vi "GetInt8.vi"(8 "error in (no error)":errorcluster, 11 "MsgPackDeserializer in":refnum<class "MsgPackDeserializer.lvclass">) -> (0 "error out":errorcluster, 2 "Number":i8, 3 "MsgPackDeserializer out":refnum<class "MsgPackDeserializer.lvclass">)   [LabVIEW 2015, in "MsgPackDeserializer.lvclass"]
uses:
  MsgPackDeserializer.lvclass
  MsgPackDeserializer.lvclass/MsgPackDeserializer.ctl
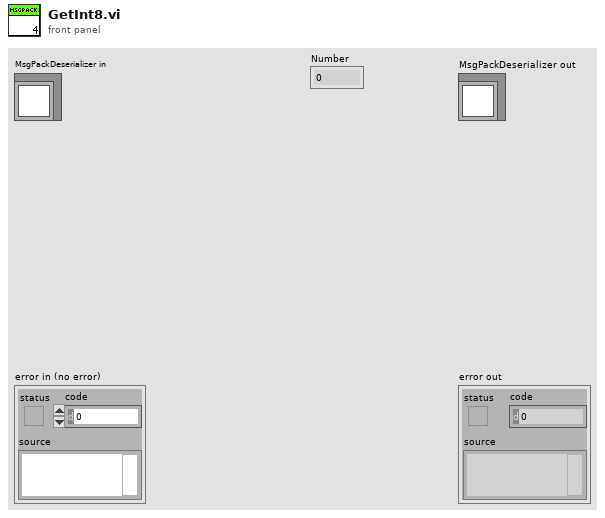
[diagram p1: front panel]
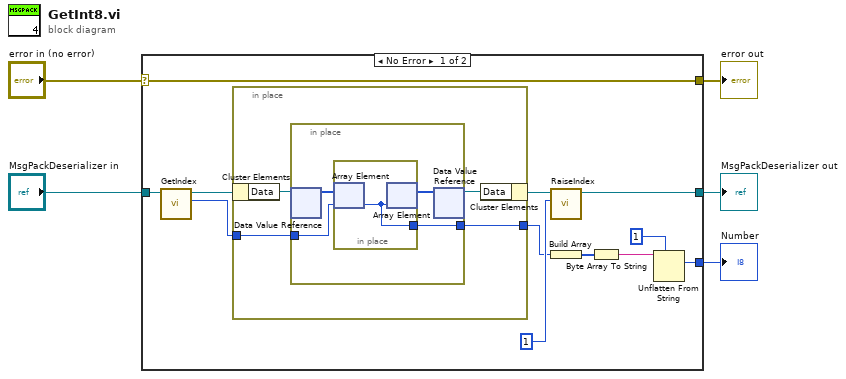
[diagram p0: block diagram]
diagram:
  n1 = case shown="No Error" "error in (no error)" {
    selector: "error in (no error)" -> [w17 w28]
    tunnel: [w17 w28] -> w4
    tunnel: [w13 w27] -> w2
    tunnel: "MsgPackDeserializer in" -> [w16 w27]
    tunnel: [w6 _] -> w1
    frame No Error {
      n2 = call "GetIndex.vi"("MsgPackDeserializer in"=w16) -> ("Index"=w14:i64, "MsgPackDeserializer out"=w15:refnum<class "MsgPackDeserializer.lvclass">)  [unwired: 8 in, 1 out]
      n3 = in-place {
        in-place-border: [w20] -> w10
        in-place-border: w14 -> [w19]
        n4 = in-place-cluster #1(w15) -> ("Data"=w18:refnum<data-value>)
        n5 = in-place {
          in-place-border: [w25] -> w20
          in-place-border: w19 -> [w24]
          n6 = in-place-dvr #2(w18) -> (w23:u8[])  [unwired: 1 out]
          n7 = in-place {
            in-place-border: [w26] -> w25
            n8 = in-place-array #3(w23, w24) -> (w26:u8)
            n9 = in-place-array #3(w26) -> (w22:u8[])  [unwired: 1 out]
          }
          n10 = in-place-dvr #2(w22) -> (w21:refnum<data-value>)  [unwired: 1 out]
        }
        n11 = in-place-cluster #1("Data"=w21) -> (w12:refnum<class "MsgPackDeserializer.lvclass">)
      }
      n12 = call "RaiseIndex.vi"("x"=i64 1, "MsgPackDeserializer in"=w12) -> ("MsgPackDeserializer out"=w13:refnum<class "MsgPackDeserializer.lvclass">)  [unwired: 8 in, 1 out]
      n13 = Build Array(w10) -> (w9:u8[])
      n14 = Byte Array To String(unsigned byte array=w9) -> (string=w8:string)
      n15 = Unflatten From String(type=i8 1 ("x"), binary string=w8) -> (value=w6:i8)  [unwired: 3 in, 2 out]
    }
    frame Error {
    }
  }
  "error out" <- w4
  "MsgPackDeserializer out" <- w2
  "Number" <- w1
